vi "Event_Counter.vi"(10 "input":bool) -> (2 "Counts":u32)   [LabVIEW 2014]
panel:
  # "U32 counter, zeroed at first call"
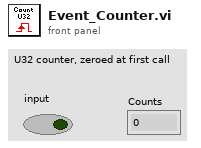
[diagram p1: front panel]
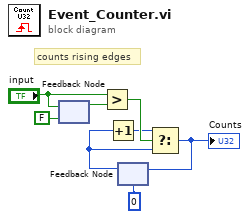
[diagram p0: block diagram]
diagram:
  # "counts rising edges"
  n1 = feedback-in #1("input") -> ()
  n2 = feedback #1(FALSE ("input")) -> (w2:bool)
  n3 = Greater?(x="input", y=w2) -> (0:w8:bool)
  n4 = feedback #2(u32 0) -> (w5:u32)
  n5 = Increment(x=w5) -> (x+1=w7:u32)
  n6 = Select(t=w7, s=w8, f=w5) -> (s? t:f=w4:u32)
  "Counts" <- w4
  n7 = feedback-in #2(w4) -> ()
